vi "2023_day03.vi"() -> ()   [LabVIEW 2021]
uses:
  <userlib>/_OpenG.lib/array/array.llb/Sort 2D Array (I32)__ogtk.vi
panel:
  out "Task 2":i32
  out "Task 1":i32
  in  "Switch":bool caption="Ex. Data  vs.  User Data"
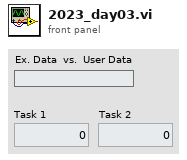
[diagram p1: front panel]
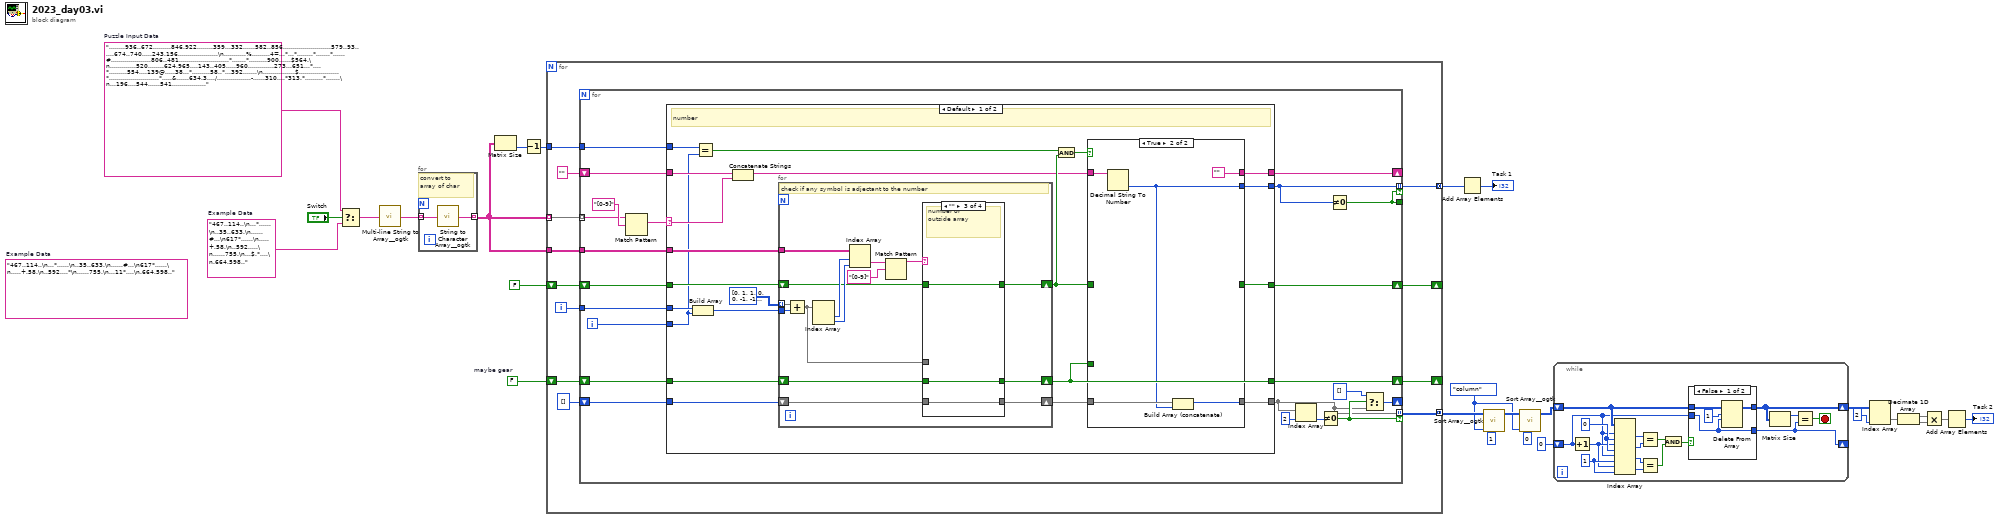
[diagram p0: block diagram]
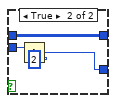
[diagram p2: hidden frame]
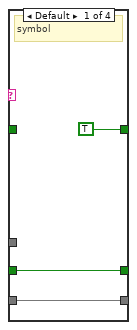
[diagram p4: hidden frame]
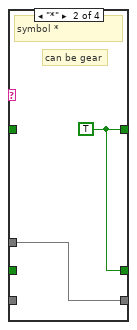
[diagram p5: hidden frame]
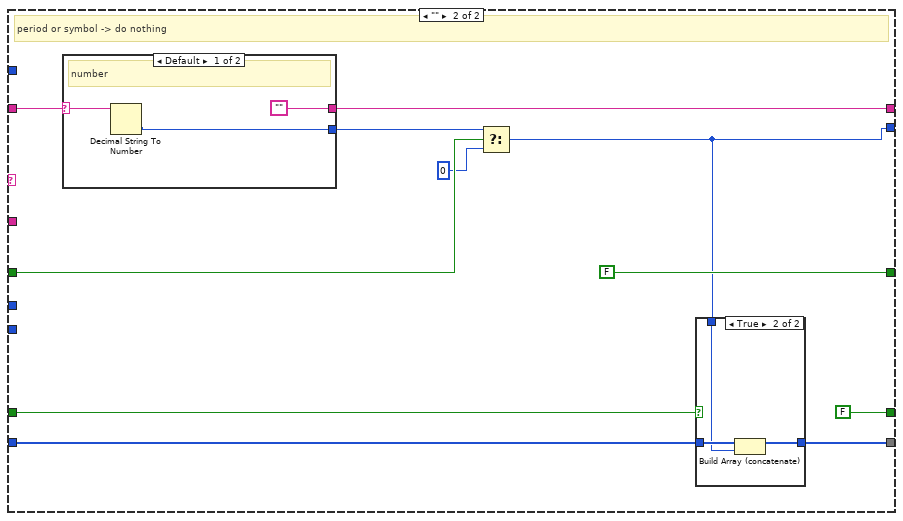
[diagram p7: hidden frame]
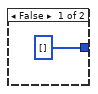
[diagram p8: hidden frame]
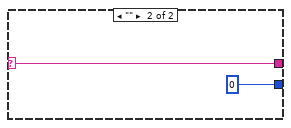
[diagram p9: hidden frame]
diagram:
  w10 = enum16{"row", "column"}."column" ("Sort By in")
  (unwired) "467..114..\n...*......\n..35..633.\n......#...\n617*......\n.....+.58.\n..592....*\n......755.\n...11*....\n.664.598.."  # Example Data
  w16 = FALSE  # maybe gear
  w25 = "........936..672.........846.922........359...332......582..856........................579..93......674..740.....243.156....................\n...........%.........4=...*...*........*.......*......#....................806..481.........................*.......*.........900......$564.\n.............520........624.965....143..405.....960.............273...651...*....*.........554....139@.....38...*.........58..*...392.......\n................$....................*.........................*.....&......634.3..../.................-......310....*313.*.........*.......\n...196....544......541................775.216...+557..225/..463.......................517..........960.228........452.....593.......772.....\n.....*....*...654.*........638............*...........................163....................386#......................20......169..........\n.....566..20...$...132........*969......747........*971..342............=.245*.......................277.522............*..............+....\n.............+..............................205.716...........................855.............324......................871..752.........291.\n.........47..390.......128...%....528........%..........91*192.......=.....................=.#.............%..852*156......+................\n.....975..*.......=....*...322.......#............&63.............946...................462....939..520...268............#.....*....380.....\n.........55..=.....871..68.............................................491.......................*.....*............674.770.333.415...*.275.\n..............633...........@.....642.5........+.......739........632.....*.......992.74.615...858...998.............*..............761.*...\n....446......................180./..../........83...&.....*924....&........379...*......................................................118.\n...........488*240.......150......................958..........$.....&...........964...351...........+..633.........123....../603...........\n...................987....../........546-...674...............466.....602.............@...........956..#............./......................\n......503=....465.................91.........*..........................................583..............128..124..........$.....217........\n..............*...32$..53....&594.........648...827....*..994.......971...................*..........304...%....*.......387..80.............\n............756.......#..........................*..888...$............@....339.......+..868........*........851..............*.........128.\n...905-.........312..................729...356*.697.........736.....+.......+.......748.......797....41....................272..753.........\n.................*....&604............*.............%915.......*.529..889...................*.........................992.........*.....718.\n...........272....487..............+...961.892..............632........*.................502.118....141................@......546.669.......\n787..........*....................85............/..330...........-...374.............................*.........446...%.........*............\n....-...../...120....919&.....................339....*....*663...403........167...533.170.............698..587...*....279.......776.+.......\n.575.....34.*.................668...19..759.......804..730...../.............*...........*.....789...........*....803......666.......25.....\n............375...773*.............*.........................$.876...287......201........484......*.........196.............................\n565...866.............23..477...455....................794.996.........*.....................887.959...146...........496....790.............\n..............648...........+........325.738....156.....*.........534..941.....%536..31..../.%...........*............*.....*.......511.....\n..............*.................166.....*......*.....647..........*......................262...........887..210.3..860.....161....4....*420.\n......141.606...........193.111..*..........252......................935*689..................500...........*...*.................*.........\n..635....*........=........*.....959.....................@834.................-.....542..547....-..........770.8...........439..............\n.................896.........93......................244..........@......247..735..*.................................497.............%......\n...............................%........................*..........200....+.......342.613.245.@............$.........#....*.......176...21..\n......51......702.37.......798....325.....&974.....834.860.....+.........................*.....533..866....864.............269..............\n..141..*......................-...&............875*.............207...882*.........................*............309.739........%......../...\n.......394....144.....................................$...................835.3..........290.......489...........&.....*177.833....866$.153.\n.689.................719.314/..$......673.....5*557...443......+..#649.............575....*..634*...........................................\n....&...........794...*........614...*......................350.............411......*.104.......141........369...934...........997.........\n.......519......*...787..............739.....628...................................784.......$..........989*........*...987.......*....#....\n.........*...309.........209.............957*........50.....@995...765.......269.@........380..624.................643.....*....836...356...\n......886............234.+....................51*935..*...........*.....188.......73..............*696...14.....#...........................\n............203..948...&...............................957......804.736*......388....689.219*660........*.....218....................$..40..\n..............*.....*.....475.....930..........%................................*......*..............477.624................848...687......\n....57*.50.229....636....*.................804.164....590.........-....547..80..310....675.......=.@...........................*............\n........................398......&........*..............*.....748...........*................226..200................160......853..........\n......292........................889.......867.....365...............192+..530.........................@910....=..222*.............894......\n..427....#.../...959........................................322.....................735*304....742..........195..........$..............22..\n...........465..-.........52.$......168.......418.......+.........................................$..............&......563...649*26........\n....................464..../.969....*......-..*........150......724.....83..301...............527...............858.506.....................\n...935.........910....+...........116....427...347.............-........*.....=.......891.......*....847...750........@................531..\n....*.........$.........676...............................510............11.......647.*.................#.....%.683.............193...+.....\n....761.169...............=...524........&......152..........*...975.994.........*....122..........858*...........%.......776...........*...\n...........-..180/.850..............$.....524....-...........940.=......*......199........963..............#........836...*.....34...543.448\n482...947...................94&....541..............265..............477..890..............*....988.....343..........&...599....+...........\n.......*...532..81..73..417............992/...99&...#........................*.33@.149..305.........678.....31.........@.................417\n....304.....@.....*...#../....452.842.................519.....307.949.....268................=.........*....*...........259.................\n..................361............*.......346............*.+......*...........................288.......492..985.............727.683.........\n....530....438..........950..........*......*........787..316...............762.724.257..889.....................844.......*......=....@125.\n..............*...446...*......879..827......148......................*730.......@..........*...832...............*.......647.......48......\n....500.......994........41.......*.....#805...........*...........614...............*....940................291&.129.8............=........\n....*...#..........698..........581.................940.462.....@......443...82.784.593......../.#375..%148............*..#.................\n.....39.562...784............................................805...$......@...*..*..........844.....................776....363...667........\n................%...265.......337.....438...295.....................499......341.74..................271.405.......................%.155....\n.........97..........*......@....*252.*......*....+.........270.229.................394...879*247.....*...*.....146.....................*...\n........%.............226..258........996.944......793........*.../...................+..............321.578.....$..........838.....529.831.\n.................%109.........................................615....822.....................501.............616....293.....&........-......\n.......%....482...........................%717.236.......562...........*...........915...580....*............*.....+..........230...........\n.....303.......*128..86&......762.928.............$........*......861*.311........*....../....517..........471.544.....996.......*38...628..\n...........563............89.*......*.583...%.148.......$.987...................35..................996...........=....*...............*....\n......776.....+...........*......967...@..168...*.....772.........838*.....480..............................-........976..............530...\n................649*32...84.#...................315...................37............398.656...631..........340.985*..........522............\n............................922........................./.173....894................*.........$....................177.......#..............\n......................................................423....*....*.....816.........13.................=..............................251...\n..154...................878*......................568......723..329....&......928.................-71.123.378..100...................*......\n........*21..250............448.734.718.....&....*......................................599...............%....*.....700+.....*803..401.....\n.779.550........*.817............./..*....118....980..589.....235......=....539...........*...281*236..........591.........927..........*...\n...-.................*...............854.............*.................911.=............939........................616..*............770.50.\n.............82......399.......452..................184........643..........................*871..................*....370..................\n.185.405.....*...634............*......189.838.................*...............@623......252...........315.86.....568...........157.104.....\n...&......586.......*........957..........*.......841.........509.600........................896..565.....*...............+............*....\n..................633.628...........811..........*.....677.........-..580..751...183.........................540.81.......656..665..634.....\n......112.............*.....=........./.322...430.........*..........+.....*...............683............$.....*...........................\n830&...*..426........649..910...........*................717..359........831........=..157..%.............143......758................579...\n.....373....*..................215.......666....................*.#...........459..547...+.........773.........980*.........404...126.......\n205......636....................*...420.......440..........225.11.516...568....*......................*....474........620...*.....*.........\n..............250......685...209.....+...........*257.................../...407.......295..498....122.............970...@.392.412...........\n783..83+...........706....=.................330*............833.................*250....%..=..........%...........*............#....898.....\n...........$....................................398..35........*......646....759.....#.............527..........160.....254.................\n500........777...........112..428...663....957#..............524.....*..../........249..530*672............567......*......*759.....284*....\n....861....................*.*......*............*...277*832.....644.130..216.446............................*...683.955................950.\n....*........826..........68.535..192.........306..................#..................762%...%....#631..500.406..........763...137..........\n..65............-...499=..................546.....&.........$........../..........177........988.......@.............336...*..*.............\n.....362..................@...$..........-....610..65......64.........830..........-...........................452......+.604.542...........\n........*902.633*........873..63.....781...31...*.................258.....12...681..........18*........&...&............................848.\n..803............752.........................-.....672...................*.............................470..86.59.......%...................\n.......@..547..........$...184.......320..........+..........471......834...=...551..108.............................176.................82.\n..950.562............261...$.....754..+..............134.654*...............778..&......%..713.837.......................329........186.....\n............112..72...............*..........917......*.................415............................946....=....614.....*................\n..............*.$......850.....766.....308.....*....666................*......812.....293................*.624.......%..296.....612...333...\n..996......154...........................*......283.....*.555.%........................-.......552.714.563.......227..............-.........\n....*.682.................=.......281.217..............84.*....908.....@...=....522..............$.*.......630......*79..............556....\n..635...*............516...402............................333........114..496..*.......324..........522.....................................\n.........511....779...*............@............350.853.........................791...................................$.....821.....+.......\n.................*.....486........984......332.....*..............893..730*480...................756...................776...........155....\n......161......57..590....................@....398..................*....................477.....*......602....506............996...........\n.151.....*..=.......*......955.......916........#.....=..269.........423..........289......*..379...*..@.....................*..............\n...-....123..927.600...........-........*395........226./....676*755...........30..........58.....582.........671.118..43.367...943......478\n.....................725........74...............................................+...........................-......*..*................&...\n........378......563*.....*999............*...................497.349...26.....$............362.........&........723....20....717...317.....\n...*....................22.........../.575.552..........291......*..........600......152.../......./...169......................-.@....*977.\n886.250..........$.............383.603.............36*.../....%......................*.............253........215..........139....583.......\n................225............................................721...814..............829..................*.......613*544.*...=........901.\n..........741.......595.........785.............%677..50................=.................252......710....91...............912.180..........\n...........*...................*....808...956..........+.....812...............*381......*.....676.../..........599....................+....\n............134.184......759..81...*.........*.782........41*......=....125.216........679...../..........@........*.................567....\n.......165.........*......@................66...*.....*.........379.....................................&..626...241........................\n.........*.........232.........387.86...........635.47.806.857.........$537...............240........617..............806..941..........531.\n.......687...654.......735......*...$......................%.....357..............*884.......*571..........273.551......*.....*....576..*...\n............*................648...................716.304..........*...690....663.................*38...........*....365......911....@..424\n....67*156...250..828...................&222.......#...*......16....300.+..................-....-.9....813...982..443.......................\n.....................*......136..757..................65..314...*........................615.291.......&....*................972............\n................721..592...@.............................../...808.............665...176.............................200.....*..............\n..198..459+............................218........-772..............169...39..*........*........939..742......#....=......532...#..264......\n.....*...............$..........713...*............................*.....*...831....689...589*.......*.......91....75.........641...#.......\n..896..167*........372...138...........462...*227..$.....801......512.........................775.673.......................................\n...............47........*.......135...............725.....*...............743..........489*.............735..622.815.551...........519.....\n.......=........*......636.987...*...................................827........496*........48.121................*.....*........#.....*311.\n....525.......819.580.........#.369......119...............77.........*...............10*........*.%.....975.....961....888......304........\n........................96*..........................816............857......=...........376...859.522..=...................................\n629...419..259...#360.......44%.........190..=969...........=...539.....-913.429......................................119.....476...707.....\n...*.....*...*....................*906.*.....................84.....286...............$...=...127.200.465........324.............=.....*599.\n905.....762...262.....-597.....847......311......@654...837............*....455..37..439..147....*.....*...262...*.....787..778.............\n...........................25...........................=...........908....*.......*................827......%....567....-....#.427..819....\n..............................#.$....643=...............................886......243....../.....672..............................*....*.....\n...........185*....107.....226..965........$.................756........................808.221...-.../574...541&...+....871...326....349...\n......................*.....................841.....=...........*688........177................*....................166....*................\n.......189..744......308.......99*391..630/........463......................@...930..........543..........................519...............\n..984.%........-.741.......................................522.915+.....769......*................207....976.....158*.......................\n....*...............*...............&.331...787........48...........224..*......184........874.......=.....*........................537.....\n.....934....*339...829....495.....682...*.............*....+..........*..794..........-430...*....&........848..367....+............*....505\n.........175..........................381............270....198......911...................52......642...............45............445......"  # Puzzle Input Data
  w14 = "467..114..\n...*......\n..35..633.\n......#...\n617*......\n.....+.58.\n..592.....\n......755.\n...$.*....\n.664.598.."  # Example Data
  n1 = Select(t=w25, s="Switch", f=w14) -> (s? t:f=w24:string)
  n2 = call <userlib>:"Multi-line String to Array__ogtk.vi"("string"=w24) -> ("lines"=w23:string[])
  n3 = for {
    tunnel: w23 -> [w28] mode=indexing
    tunnel: [w27] -> w19 mode=indexing
    # "convert to array of char"
    n4 = call <userlib>:"String to Character Array__ogtk.vi"("Input String"=w28) -> ("Character Array"=w27:string[])
  }
  n5 = Matrix Size(0:w19) -> (2:w18:i32)  [unwired: 1 out]
  n6 = Decrement(x=w18) -> (x-1=w17:i32)
  n7 = for {
    tunnel: w19 -> [w39] mode=indexing
    shift-right: [w37] -> _
    shift-left: FALSE -> [w36]
    tunnel: w19 -> [w35]
    tunnel: [w34] -> w20 mode=concatenating
    tunnel: w17 -> [w33]
    shift-right: [w32] -> _
    shift-left: w16 -> [w31]
    tunnel: [w29] -> w13 mode=concatenating
    i -> [w38]
    n8 = for {
      tunnel: w39 -> [w60] mode=indexing
      shift-right: [w58] -> _
      shift-left: "" -> [w59]
      tunnel: w38 -> [w57]
      shift-right: [w55] -> w37
      shift-left: w36 -> [w54]
      tunnel: w35 -> [w53]
      tunnel: [w51] -> w34 mode=indexing if=w52
      tunnel: [w52] -> _
      tunnel: w33 -> [w50]
      shift-right: [w41] -> _
      shift-left: i32[] [] -> [w49]
      shift-right: [w48] -> w32
      shift-left: w31 -> [w47]
      tunnel: [w43] -> w29 mode=indexing if=w44
      i -> [w56]
      n9 = Match Pattern(string=w60, regular expression="[0-9]") -> (match substring=w61:string)  [unwired: 1 in, 3 out]
      n10 = case shown="Default" w61 {
        selector: w61 -> [w82 _]
        tunnel: w59 -> [w83 w128]
        tunnel: [w71 w127] -> w58
        tunnel: w57 -> [w79 _]
        tunnel: w56 -> [w75 _]
        tunnel: [w70 FALSE] -> w55
        tunnel: w54 -> [w77 w126]
        tunnel: w53 -> [w78 _]
        tunnel: [w72 w120] -> w51
        tunnel: w50 -> [w76 _]
        tunnel: w49 -> [w68 w122]
        tunnel: [w65 w121] -> w43
        tunnel: w47 -> [w67 w118]
        tunnel: [w66 FALSE] -> w48
        frame Default {
          # "number"
          n11 = Build Array(w79, w75) -> (w80:i32[])
          n12 = Equal?(x=w76, y=w75) -> (x = y?=w74:bool)
          n13 = Concatenate Strings(w83, w82) -> (w63:string)
          n14 = for {
            tunnel: i32[][] [[0, 1], [1, 0], [0, -1], [-1, 0], [-1, 1], [-1, -1], [1, -1], [1, 1]] -> [w106] mode=indexing
            tunnel: w80 -> [w105]
            tunnel: w78 -> [w102]
            shift-right: [w97] -> w69
            shift-left: w77 -> [w98]
            shift-right: [w96] -> w64
            shift-left: w68 -> [w95]
            shift-right: [w93] -> w66
            shift-left: w67 -> [w94]
            # "check if any symbol is adjectant to the number"
            n15 = Add(x=w106, y=w105) -> (x+y=w92:i32[])
            n16 = Index Array(array=w92) -> (element #1=w104:i32, element #2=w103:i32)  [unwired: 2 in]
            n17 = Index Array(array=w102, index (row)=w104, index (col)=w103) -> (element=w100:string)
            n18 = Match Pattern(string=w100, regular expression="[0-9]") -> (before substring=w99:string)  [unwired: 1 in, 3 out]
            n19 = case shown="\"\"" w99 {
              tunnel: w98 -> [_ _ w114 w117]
              tunnel: [TRUE w111 w114 w117] -> w97
              tunnel: [w107 w110 w112 w115] -> w96
              tunnel: w95 -> [w107 _ w112 w115]
              tunnel: [w108 w111 w113 w116] -> w93
              tunnel: w94 -> [w108 _ w113 w116]
              tunnel: w92 -> [_ w110 _ _]
              frame Default {
                # "symbol"
              }
              frame "*" {
                w111 = TRUE
                # "can be gear"
                # "symbol *"
              }
              frame "" {
                # "number or\noutside array"
              }
              frame "." {
                # "period"
              }
            }
          }
          n20 = And(x=w74, y=w69) -> (x .and. y?=w73:bool)
          n21 = case shown="True" w73 {
            tunnel: w63 -> [w86 w91]
            tunnel: [_ w87] -> w72
            tunnel: [w86 ""] -> w71
            tunnel: [w85 _] -> w70
            tunnel: w69 -> [w85 _]
            tunnel: w66 -> [_ _]
            tunnel: [w84 w89] -> w65
            tunnel: w64 -> [w84 w88]
            frame False {
            }
            frame True {
              n22 = Decimal String To Number(string=w91) -> (number=w87:i32)  [unwired: 2 in, 1 out]
              n23 = Build Array (concatenate)(w88, w87) -> (w89:i32[])
            }
          }
        }
        frame "" {
          # "period or symbol -> do nothing"
          n24 = case shown="Default" w128 {
            selector: w128 -> [w135 w137]
            tunnel: ["" w137] -> w127
            tunnel: [w133 0] -> w123
            frame Default {
              # "number"
              n25 = Decimal String To Number(string=w135) -> (number=w133:i32)  [unwired: 2 in, 1 out]
            }
            frame "" {
            }
          }
          n26 = Select(t=w123, s=w126, f=0) -> (s? t:f=w120:i32)
          n27 = case shown="True" w118 {
            tunnel: [i32[] [] w131] -> w121
            tunnel: w122 -> [_ w132]
            tunnel: w120 -> [_ w130]
            frame False {
            }
            frame True {
              n28 = Build Array (concatenate)(w132, w130) -> (w131:i32[])
            }
          }
        }
      }
      n29 = Index Array(array=w43, index=2) -> (element=w46:i32)
      n30 = Not Equal To 0?(x=w46) -> (x != 0?=w44:bool)
      n31 = Not Equal To 0?(x=w51) -> (x != 0?=w52:bool)
      n32 = Select(t=i32[] [], s=w44, f=w43) -> (s? t:f=w41:i32[])
    }
  }
  n33 = Add Array Elements(numeric array=w20) -> (sum=→"Task 1":i32)
  n34 = call-poly <userlib>:"Sort Array__ogtk.vi"("Column/Row to Sort By"=u32 1, "Sort By in"=w10, "Array in"=w13) -> ("Sorted Array out"=w11:i32[][])  [unwired: 5 in, 3 out]
  n35 = call-poly <userlib>:"Sort Array__ogtk.vi"("Column/Row to Sort By"=u32 0, "Sort By in"=w10, "Array in"=w11) -> ("Sorted Array out"=w5:i32[][])  [unwired: 5 in, 3 out]
  n36 = while {
    shift-right: [w141] -> w3
    shift-left: w5 -> [w143]
    shift-right: [w140] -> _
    shift-left: 0 ("disabled index (col)") -> [w142]
    stop <- w138 stop-if-true
    w153 = 1 ("index (col)")
    w152 = 0 ("disabled index (col)")
    n37 = Increment(x=w142) -> (x+1=w151:i32)
    n38 = Index Array(array=w143, index (row) #1=w142, index (col) #1=w152, index (row) #2=w151, index (col) #2=w152, index (row) #3=w142, index (col) #3=w153, index (row) #4=w151, index (col) #4=w153) -> (element #1=w149:i32, element #2=w150:i32, element #3=w148:i32, element #4=w147:i32)
    n39 = Equal?(x=w149, y=w150) -> (x = y?=w146:bool)
    n40 = Equal?(x=w148, y=w147) -> (x = y?=w145:bool)
    n41 = And(x=w146, y=w145) -> (x .and. y?=w144:bool)
    n42 = case shown="False" w144 {
      tunnel: w143 -> [w157 w161]
      tunnel: [w156 w161] -> w141
      tunnel: w142 -> [w154 w160]
      tunnel: [w154 w159] -> w140
      frame False {
        n43 = Delete From Array(array=w157, length=1, index (row)=w154) -> (array with subset deleted=w156:i32[][])  [unwired: 1 in, 1 out]
      }
      frame True {
        n44 = Add(x=w160, y=2) -> (x+y=w159:i32)
      }
    }
    n45 = Matrix Size(0:w141) -> (1:w139:i32)  [unwired: 1 out]
    n46 = Equal?(x=w139, y=w140) -> (x = y?=w138:bool)
  }
  n47 = Index Array(array=w3, index (col)=2 ("disabled index (col)")) -> (element=w2:i32[])  [unwired: 1 in]
  n48 = Decimate 1D Array(w2) -> (w8:i32[], w7:i32[])
  n49 = Multiply(x=w8, y=w7) -> (x*y=w6:i32[])
  n50 = Add Array Elements(numeric array=w6) -> (sum=→"Task 2":i32)
